vi "Board_Colors.vi"() -> ()   [LabVIEW 2021]
panel:
  in  "Background":u32(colorbox)=7115403
  in  "Snake Body":u32(colorbox)=6618880
  in  "Snake Head":u32(colorbox)=1985280
  in  "Food":u32(colorbox)=16711680
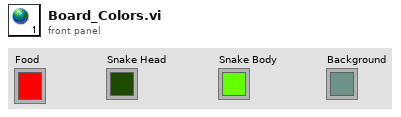
[diagram p1: front panel]
diagram:
